vi "Sub Update Frame Num.vi"(8 "error in (no error)":errorcluster, 11 "Pic Json Generator in":refnum<class "Pic Json Generator.lvclass">) -> (0 "error out":errorcluster, 3 "Pic Json Generator out":refnum<class "Pic Json Generator.lvclass">)   [LabVIEW 2018, in "Pic Json Generator.lvlib" / "Pic Json Generator.lvclass"]
uses:
  Pic Json Generator.lvclass
  Pic Json Generator.lvclass/Pic Json Generator.ctl
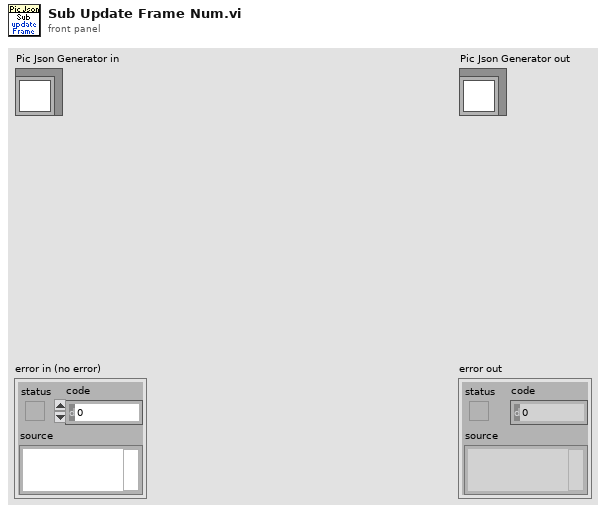
[diagram p1: front panel]
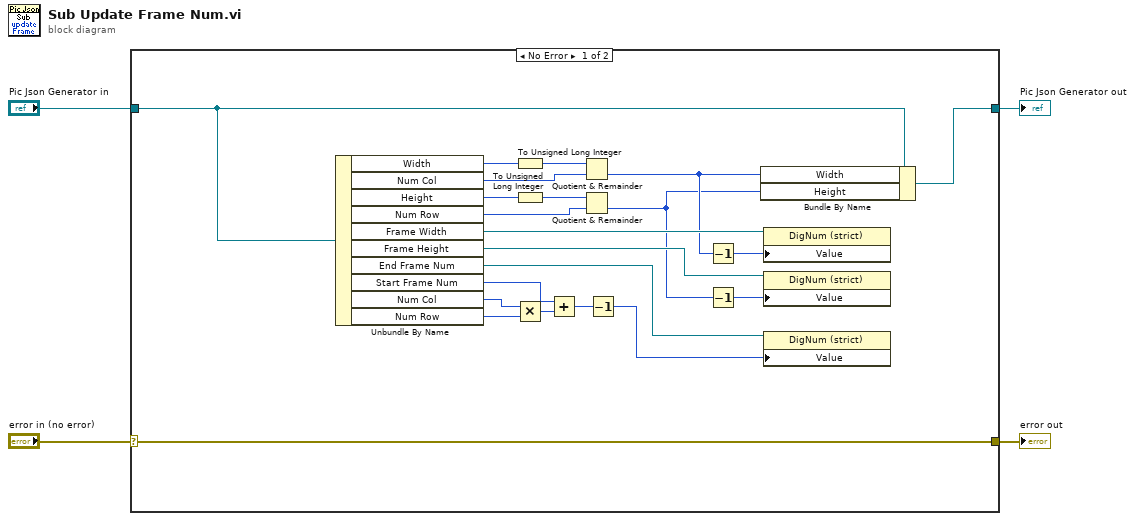
[diagram p0: block diagram]
diagram:
  n1 = case shown="No Error" "error in (no error)" {
    selector: "error in (no error)" -> [w9 w28]
    tunnel: [w9 w28] -> w3
    tunnel: [w19 w27] -> w1
    tunnel: "Pic Json Generator in" -> [w26 w27]
    frame No Error {
      n2 = Unbundle By Name(w26) -> ("Width"=w25:i16, "Num Col"=w24:u32, "Height"=w22:i16, "Num Row"=w20:u32, "Frame Width"=w18:refnum<vi>, "Frame Height"=w16:refnum<vi>, "End Frame Num"=w14:refnum<vi>, "Start Frame Num"=w8:u32, "Num Col"=w13:u32, "Num Row"=w12:u32)
      n3 = To Unsigned Long Integer(number=w25) -> (unsigned 32bit integer=w23:u32)
      n4 = To Unsigned Long Integer(number=w22) -> (unsigned 32bit integer=w21:u32)
      n5 = Multiply(x=w13, y=w12) -> (x*y=w11:u32)
      n6 = Add(x=w8, y=w11) -> (x+y=w10:u32)
      n7 = Quotient & Remainder(x=w23, y=w24) -> (floor(x/y)=w17:u32)  [unwired: 1 out]
      n8 = Quotient & Remainder(x=w21, y=w20) -> (floor(x/y)=w15:u32)  [unwired: 1 out]
      n9 = Decrement(x=w10) -> (x-1=w7:u32)
      n10 = Decrement(x=w17) -> (x-1=w6:u32)
      n11 = Decrement(x=w15) -> (x-1=w5:u32)
      n12 = Bundle By Name(cluster=w26, "Width"=w17, "Height"=w15) -> (w19:refnum<class "Pic Json Generator.lvclass">)
      n13 = property class="DigNum (strict)"(reference=w18, "Value"=w6) -> ()  [unwired: 1 in, 2 out]
      n14 = property class="DigNum (strict)"(reference=w16, "Value"=w5) -> ()  [unwired: 1 in, 2 out]
      n15 = property class="DigNum (strict)"(reference=w14, "Value"=w7) -> ()  [unwired: 1 in, 2 out]
    }
    frame Error {
    }
  }
  "error out" <- w3
  "Pic Json Generator out" <- w1
